vi "Test GraphLockin_vs_Parameter.vi"() -> ()   [LabVIEW 2016]
uses:
  <userlib>/_OpenG.lib/numeric/numeric.llb/Random Number Within Range - I32__ogtk.vi
  src/Transport/Transport.lvclass
panel:
  out "time vs parameter":cluster{i32[], u32[]}(graph)
  out "ms":u32
  out "G(Siemens) vs Parameter":cluster{"Y":dbl[], "Y":dbl[]}[](graph)
  in  "V2":i32=1 min=1
  in  "V1":i32=1 min=1
  in  "Current":i32=1 min=1
  out "X vs Parameter":cluster{dbl[], dbl[]}[](graph)
  in  "reset?":bool
  in  "stop":bool
  # "try changing these:"
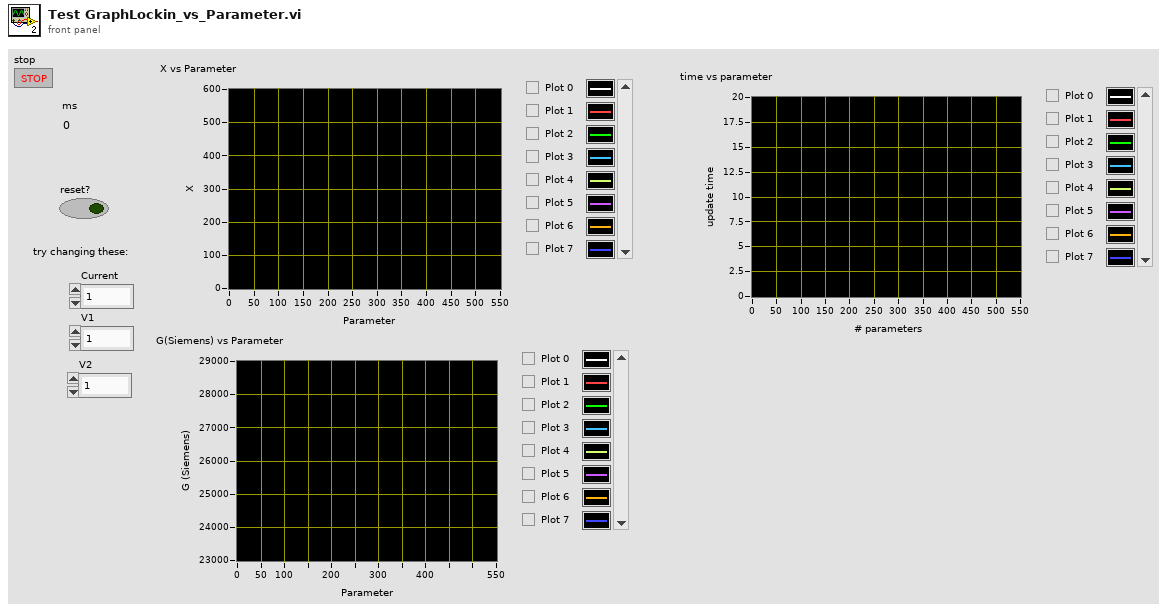
[diagram p1: front panel]
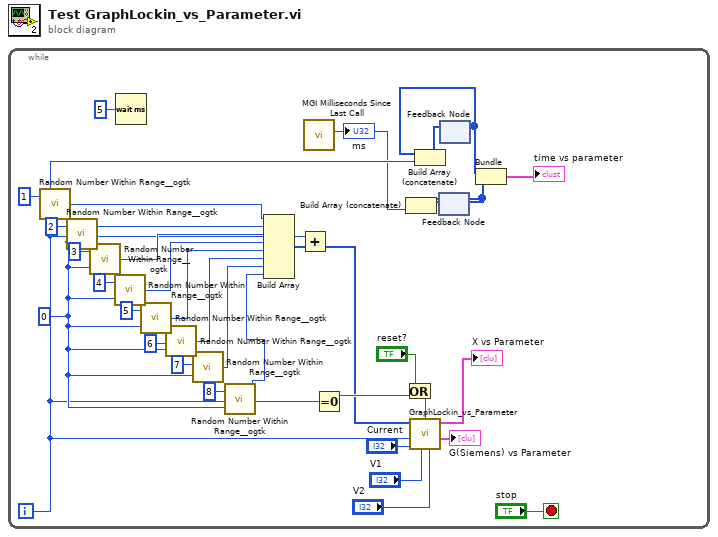
[diagram p0: block diagram]
diagram:
  n1 = while {
    i -> [w7]
    stop <- "stop" stop-if-true
    w35 = 0 ("Low")
    n2 = call-poly <userlib>:"Random Number Within Range__ogtk.vi"("High"=1, "Low"=w35) -> ("Random Number"=w32:i32)  [unwired: 3 in]
    n3 = call-poly <userlib>:"Random Number Within Range__ogtk.vi"("High"=2, "Low"=w35) -> ("Random Number"=w31:i32)  [unwired: 3 in]
    n4 = call-poly <userlib>:"Random Number Within Range__ogtk.vi"("High"=3, "Low"=w35) -> ("Random Number"=w30:i32)  [unwired: 3 in]
    n5 = call-poly <userlib>:"Random Number Within Range__ogtk.vi"("High"=4, "Low"=w35) -> ("Random Number"=w29:i32)  [unwired: 3 in]
    n6 = Wait (ms)(milliseconds to wait=u32 5) -> ()  [unwired: 1 out]
    n7 = call-poly <userlib>:"Random Number Within Range__ogtk.vi"("High"=5, "Low"=w35) -> ("Random Number"=w28:i32)  [unwired: 3 in]
    n8 = call-poly <userlib>:"Random Number Within Range__ogtk.vi"("High"=6, "Low"=w35) -> ("Random Number"=w27:i32)  [unwired: 3 in]
    n9 = call-poly <userlib>:"Random Number Within Range__ogtk.vi"("High"=7, "Low"=w35) -> ("Random Number"=w26:i32)  [unwired: 3 in]
    n10 = call-poly <userlib>:"Random Number Within Range__ogtk.vi"("High"=8, "Low"=w35) -> ("Random Number"=w25:i32)  [unwired: 3 in]
    n11 = Build Array(w32, w31, w30, w29, w28, w27, w26, w25) -> (w33:i32[])
    n12 = Add(x=w7, y=w33) -> (x+y=w12:i32[])
    n13 = call <userlib>:"MGI Milliseconds Since Last Call.vi"() -> ("ms"=w4:u32)  [unwired: 6 in, 1 out]
    "ms" <- w4
    n14 = Equal To 0?(x=w7) -> (x = 0?=w13:bool)
    n15 = Or(x="reset?", y=w13) -> (x .or. y?=w14:bool)
    n16 = call "GraphLockin_vs_Parameter.vi"("V-"="V2", "V+"="V1", "reset?"=w14, "Current"="Current", "Parameter"=w7, "X[ ]"=w12) -> ("G(e2/h) vs Parameter"=→"G(Siemens) vs Parameter":cluster{"Y":dbl[], "Y":dbl[]}[], "X vs Parameter"=→"X vs Parameter":cluster{dbl[], dbl[]}[])  [unwired: 2 in, 2 out]
    n17 = feedback #1() -> (w2:u32[])  [unwired: 1 in]
    n18 = Build Array (concatenate)(w2, w4) -> (w3:u32[])
    n19 = feedback-in #1(w3) -> ()
    n20 = feedback #2() -> (w5:i32[])  [unwired: 1 in]
    n21 = Build Array (concatenate)(w5, w7) -> (w6:i32[])
    n22 = feedback-in #2(w6) -> ()
    n23 = Bundle(w5, w2) -> (→"time vs parameter":cluster{i32[], u32[]})  [unwired: 1 in]
  }
